vi "CAN Reset.vi"(8 "error in":errorcluster, 11 "Channel":u16) -> (0 "error out":errorcluster, 3 "Channel out":u16, 5 "function return":u32)   [LabVIEW 2025, in "PCAN2023.lvlib"]
doc: "Resets the receive and transmit queues of the PCAN Channel\n\n\n\nTPCANStatus __stdcall CAN_Reset(\n TPCANHandle Channel);"
uses:
  PCAN2023.lvlib
  x64/PCANBasic.dll
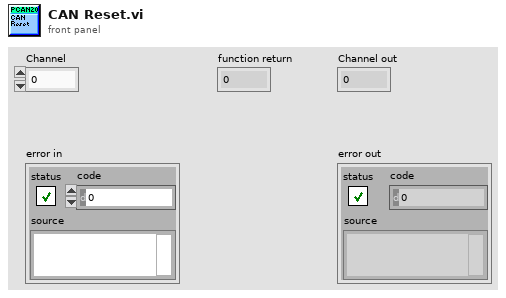
[diagram p1: front panel]
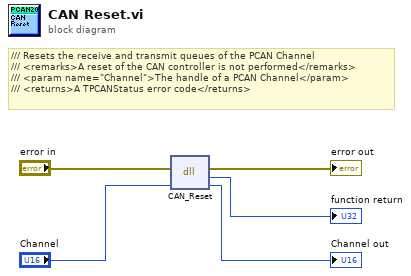
[diagram p0: block diagram]
diagram:
  # "/// Resets the receive and transmit queues of the PCAN Channel\n/// <remarks>A reset of the CAN controller is not performed</remarks>\n/// <param name=\"Channel\">The handle of a PCAN Channel</param>\n/// <returns>A TPCANStatus error code</returns>"
  n1 = dll-call lib="C:/UTP/LabView/Communication Handle/PCAN2023/x64/PCANBasic.dll" fn="CAN_Reset"(error in="error in", "Channel"="Channel") -> (error out=→"error out":errorcluster, "return type"=→"function return":u32, "Channel"=→"Channel out":u16)  [unwired: 2 in, 1 out]
